vi "Start.vi"(8 "error in (no error)":errorcluster, 11 "DIO DAQmx PWM CFG in":refnum<class "CO DAQmx PWM CFG Simulated.lvclass">) -> (0 "error out":errorcluster, 3 "DIO DAQmx PWM CFG out":refnum<class "CO DAQmx PWM CFG Simulated.lvclass">)   [LabVIEW 2024, in "DAQmx Simulated CFGs.lvlib" / "CO DAQmx PWM CFG Simulated.lvclass"]
uses:
  CO DAQmx PWM CFG Simulated.lvclass
  CO DAQmx PWM CFG/CO DAQmx PWM CFG.lvclass
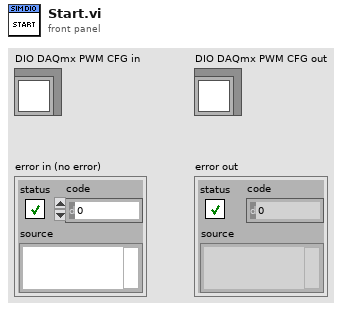
[diagram p1: front panel]
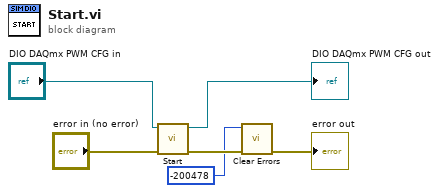
[diagram p0: block diagram]
diagram:
  n1 = call-parent "Start.vi"("error in"="error in (no error)", "DAQmx Base CFG in"="DIO DAQmx PWM CFG in") -> ("error out"=w6:errorcluster, "DAQmx Base CFG out"=→"DIO DAQmx PWM CFG out":refnum<class "CO DAQmx PWM CFG Simulated.lvclass">)  [unwired: 8 in]
  n2 = call <vilib>:"Clear Errors.vi"("error in (no error)"=w6, "specific error code to clear (0: all)"=-200478) -> ("error out"=→"error out":errorcluster)  [unwired: 4 in, 1 out]
